vi "Write Trigger.lvclass.vi"(8 "error in (no error)":errorcluster, 10 "Trigger.lvclass":refnum<class "Trigger.lvclass">, 11 "Sync Box in":refnum<class "Sync Box.lvclass">) -> (0 "error out":errorcluster, 3 "Sync Box out":refnum<class "Sync Box.lvclass">)   [LabVIEW 2012, in "Sync Box.lvclass"]
uses:
  Sync Box.lvclass
  Trigger/Trigger.lvclass
  Sync Box.lvclass/Sync Box.ctl
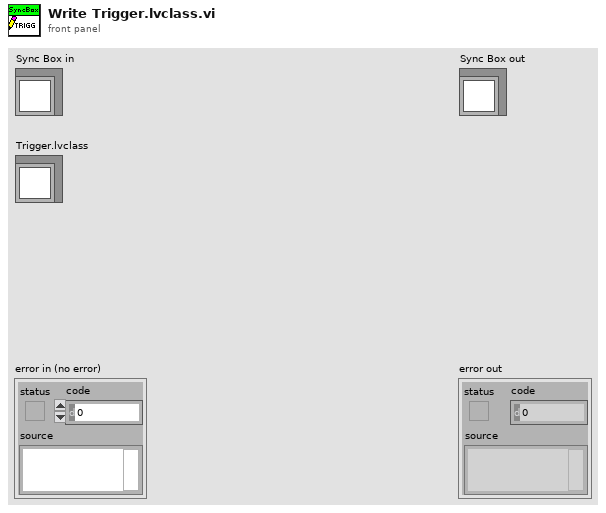
[diagram p1: front panel]
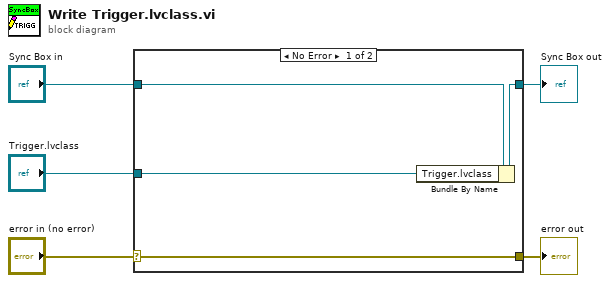
[diagram p0: block diagram]
diagram:
  n1 = case shown="No Error" "error in (no error)" {
    selector: "error in (no error)" -> [w9 w10]
    tunnel: [w9 w10] -> w4
    tunnel: [w7 w11] -> w2
    tunnel: "Sync Box in" -> [w8 w11]
    tunnel: "Trigger.lvclass" -> [w6 _]
    frame No Error {
      n2 = Bundle By Name(cluster=w8, "Trigger.lvclass"=w6) -> (w7:refnum<class "Sync Box.lvclass">)
    }
    frame Error {
    }
  }
  "error out" <- w4
  "Sync Box out" <- w2
